vi "Test Insight.vi"() -> ()   [LabVIEW 2014, in "Insight.lvclass"]
uses:
  Insight.lvclass
panel:
  out "Status":string
  out "Insite out":refnum<class "Insight.lvclass">
  out "error out":errorcluster
  in  "error in (no error) 2":errorcluster
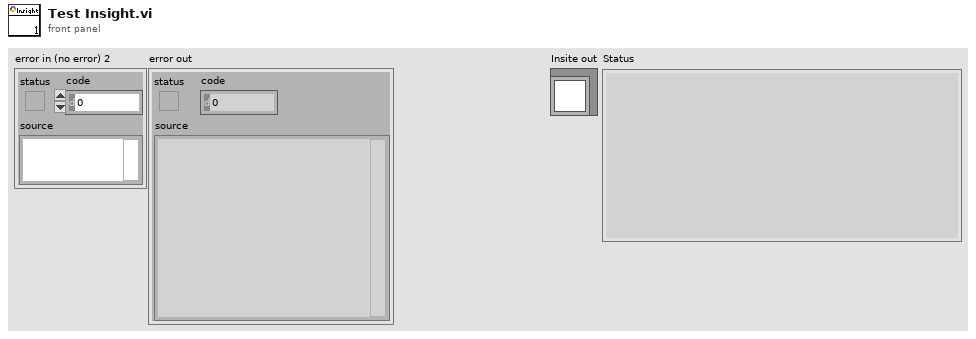
[diagram p1: front panel]
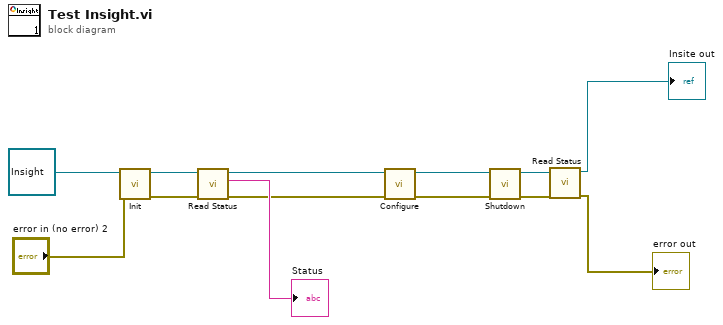
[diagram p0: block diagram]
diagram:
  n1 = call-dynamic "Init.vi"("error in (no error)"="error in (no error) 2", "Insite in"=refnum<class "Insight.lvclass"> refnum ("Insight.lvclass")) -> ("error out"=w10:errorcluster, "Insite out"=w11:refnum<class "Insight.lvclass">)  [unwired: 8 in]
  n2 = call-dynamic "Read Status.vi"("error in (no error)"=w10, "Laser in"=w11) -> ("error out"=w1:errorcluster, "Status"=→"Status":string, "Laser out"=w2:refnum<class "Insight.lvclass">)  [unwired: 7 in]
  n3 = call-dynamic "Configure.vi"("error in (no error)"=w1, "Insight in"=w2) -> ("error out"=w4:errorcluster, "Insight out"=w3:refnum<class "Insight.lvclass">)  [unwired: 8 in]
  n4 = call-dynamic "Shutdown.vi"("error in (no error)"=w4, "Insight in"=w3) -> ("error out"=w8:errorcluster, "Insight out"=w7:refnum<class "Insight.lvclass">)  [unwired: 8 in]
  n5 = call-dynamic "Read Status.vi"("error in (no error)"=w8, "Laser in"=w7) -> ("error out"=→"error out":errorcluster, "Laser out"=→"Insite out":refnum<class "Insight.lvclass">)  [unwired: 7 in, 1 out]
